vi "InitCtlRefs_Base.vi"(4 "Add Array Ctls?":bool=TRUE, 6 "Add Cluster Ctls?":bool=TRUE, 8 "error in (no error)":errorcluster, 11 "VI in":refnum<vi>) -> (0 "error out":errorcluster, 2 "Data Value Reference out":T1, 3 "VI out":refnum<vi>)   [LabVIEW 2020, in "CtlReferences.lvlib" / "CtlReferences.lvclass"]
uses:
  CtlReferences.lvclass
  TypeDefs/CtlLookup.ctl
  AddControl.vi
  CtlReferences.lvclass/CtlReferences.ctl
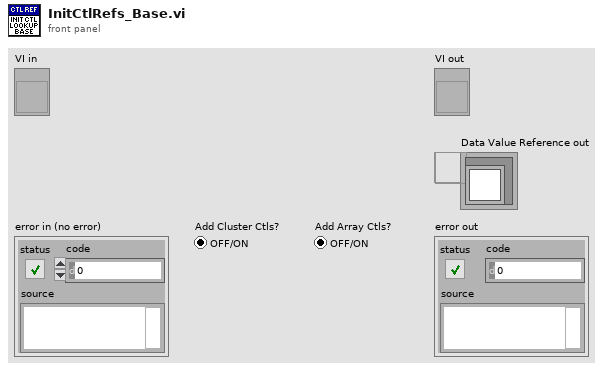
[diagram p1: front panel]
types:
  T1 = typedef "CtlReferences.lvlib/CtlReferences.lvclass/CtlLookup.ctl" = refnum<data-value>
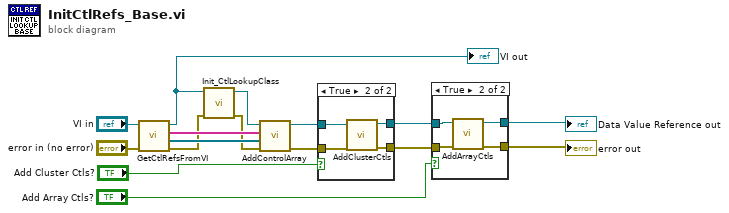
[diagram p0: block diagram]
diagram:
  n1 = call "GetCtlRefsFromVI.vi"("error in"="error in (no error)", "VI (Caller)"="VI in") -> ("error out"=w3:errorcluster, "RefArray"=w16:refnum<vi>[], "RefName Array"=w15:string[], "VI (Caller) Out"=w1:refnum<vi>)  [unwired: 6 in]
  "VI out" <- w1
  n2 = call "Init_CtlLookupClass.vi"("error in (no error)"=w3, "VIRefIn"=w1) -> ("error out"=w2:errorcluster, "CtlLookup"=w4:T1)  [unwired: 8 in]
  n3 = call "AddControlArray.vi"("error in (no error)"=w2, "CtlRef Array"=w16, "CtlLabel Array"=w15, "CtlLookup In"=w4) -> ("error out"=w12:errorcluster, "CtlLookup Out"=w11:T1)  [unwired: 6 in]
  n4 = case shown="True" "Add Cluster Ctls?" {
    tunnel: w12 -> [w17 w22]
    tunnel: w11 -> [w18 w21]
    tunnel: [w18 w20] -> w9
    tunnel: [w17 w19] -> w8
    frame False {
    }
    frame True {
      n5 = call "AddClusterCtls.vi"("error IO In"=w22, "CtlLookup In"=w21) -> ("error IO"=w19:errorcluster, "CtlLookup Out"=w20:T1)  [unwired: 8 in]
    }
  }
  n6 = case shown="True" "Add Array Ctls?" {
    tunnel: w8 -> [w23 w25]
    tunnel: w9 -> [w24 w26]
    tunnel: [w24 w27] -> w6
    tunnel: [w23 w28] -> w7
    frame False {
    }
    frame True {
      n7 = call "AddArrayCtls.vi"("error IO In"=w25, "CtlLookup In"=w26) -> ("error IO"=w28:errorcluster, "CtlLookup Out"=w27:T1)  [unwired: 8 in]
    }
  }
  "Data Value Reference out" <- w6
  "error out" <- w7
